vi "Navigation_Main_derping_stuff_up april 14.vi"() -> ()   [LabVIEW 2015]
uses:
  <vilib>/myRIO/Instrument Drivers/Onboard IO/PWM/typedefs/PWM Reference.ctl
  <vilib>/myRIO/Common/Instrument Driver Framework/Utilities/typedefs/myRIO Generic Hardware Reference.ctl
  <vilib>/myRIO/Common/Instrument Driver Framework/Utilities/typedefs/Hardware Version Enum.ctl
  <vilib>/myRIO/Common/Instrument Driver Framework/Utilities/typedefs/myRIO v1.0 Reference.ctl
  <vilib>/myRIO/Common/Instrument Driver Framework/Utilities/typedefs/Generic FPGA Reference.ctl
  <vilib>/myRIO/Common/Instrument Driver Framework/myRIO v1.0/PWM/typedefs/PWM Channels Enum.ctl
  <vilib>/myRIO/Instrument Drivers/Onboard IO/PWM/typedefs/PWM Configuration.ctl
  <vilib>/userdefined/High Color/nirio_resource_hc.ctl
  <vilib>/myRIO/Common/Instrument Driver Framework/myRIO v1.0/PWM/vis/myRIO v1.1 Open PWM.vi
  <vilib>/myRIO/Common/Instrument Driver Framework/Utilities/vis/Validate Channels.vi
  <vilib>/myRIO/Common/Instrument Driver Framework/myRIO v1.0/PWM/vis/myRIO v1.0 Reserve PWM.vi
  <vilib>/myRIO/Common/Instrument Driver Framework/myRIO v1.0/PWM/vis/myRIO v1.0 Build MUX Configuration PWM.vi
  <vilib>/myRIO/Common/Instrument Driver Framework/myRIO v1.0/Resource Manager/vis/myRIO v1.0 Reserve Channel List.vi
  <vilib>/myRIO/Common/Instrument Driver Framework/myRIO v1.0/Resource Manager/vis/myRIO v1.0 Create Configuration List.vi
  <vilib>/myRIO/Common/Instrument Driver Framework/myRIO v1.0/Resource Manager/vis/myRIO v1.0 Reserve Channel.vi
  <vilib>/myRIO/Common/Instrument Driver Framework/myRIO v1.0/Resource Manager/vis/myRIO v1.0 Unreserve Channel.vi
  <vilib>/myRIO/Common/Instrument Driver Framework/myRIO v1.0/Resource Manager/vis/myRIO v1.0 Build Mutex Name.vi
  <vilib>/FPGAPlugInAG/myRIO-1900/niLvFpga_Open_myRIO-1900.vi
  <vilib>/rvi/interface/common/dynamic/niFpgaDynamicAddResources.vi
  <vilib>/myRIO/Common/Instrument Driver Framework/Utilities/vis/FPGA Ref Manager.vi
  <vilib>/Utility/error.llb/Error Cluster From Error Code.vi
  <vilib>/myRIO/Common/Instrument Driver Framework/Utilities/vis/Ref Counter.vi
  <vilib>/rvi/errors/niLvFpgaAdjustHostInterfaceError.vi
  <vilib>/Utility/VariantDataType/GetNumericInfo.vi
  <vilib>/myRIO/Common/Instrument Driver Framework/myRIO v1.0/myRIO v1.1 Open.vi
  <vilib>/myRIO/Common/Instrument Driver Framework/Utilities/vis/IO Manager.vi
  <vilib>/myRIO/Common/Instrument Driver Framework/Utilities/vis/Configuration Manager.vi
  <vilib>/myRIO/Common/Instrument Driver Framework/myRIO v1.0/Resource Manager/vis/myRIO v1.0 Configure IO.vi
  <vilib>/myRIO/Common/Instrument Driver Framework/myRIO v1.0/myRIO v1.0 Close.vi
  <vilib>/myRIO/Common/Instrument Driver Framework/myRIO v1.0/PWM/vis/myRIO v1.0 Write PWM.vi
  <vilib>/addons/control/pid/pid.llb/PID (DBL).vi
  <vilib>/rvi/interface/nirviOpenFPGA/nirviOpenFPGA.xnode
  Navi/E/FPGA Bitfiles/NavigationProjec_FPGATarget2_FPGAMainNavigati_PWPHW8gwDxI.lvbitx
  <vilib>/rvi/interface/nirviReadWriteControl/nirviReadWriteControl.xnode
  <vilib>/myRIO/Instrument Drivers/Onboard IO/PWM/vis/myRIO PWM Open.xnode
  <vilib>/myRIO/Instrument Drivers/Onboard IO/PWM/PWM.lvlib
  <vilib>/myRIO/Instrument Drivers/Utilities/Utilities.lvlib
  NiFpgaLv.dll
  <vilib>/rvi/interface/Simulation/niFpgaSimulationCallBeginRW.vi
  <vilib>/addons/control/pid/NI_PID_pid.lvlib
panel:
  out "distance to goal":dbl
  out "loc_y":dbl
  out "loc_x":dbl
  out "loc_theta":dbl
  out "start y":dbl
  out "start angle":dbl=1.0
  out "start x":dbl=1.0
  in  "set start position":bool=TRUE
  out "goal reached":bool=TRUE
  out "x/y":dbl
  out "scale":dbl=1.0
  in  "x goal":dbl=10.0
  in  "L Desired Input Velocity (ft/s) 4":dbl(knob) scale=-4.0..4.0
  in  "R Min Linear Velocity (ft/s)  2":dbl=-2.0 format="%#_13g"
  in  "L Min Linear Velocity (ft/s) 9":dbl=-2.0 format="%#_13g"
  in  "R Max Linear Velocity (ft/s) 5":dbl=2.0 format="%#_13g"
  in  "L Max Linear Velocity (ft/s) 5":dbl=2.0 format="%#_13g"
  in  "R Desired Input Velocity (ft/s) 5":dbl(knob) scale=-4.0..4.0
  out "left":dbl
  out "right":dbl
  out "left wheels actual pwm":dbl
  in  "stop 3":bool
  out "left pwm":dbl(graph)
  out "dt out (s) 3":dbl format="%.3f"
  in  "output range 3":cluster{"output high":dbl, "output low":dbl}={"output high"=0.13333, "output low"=-0.13333} {"output low" format="%.6f"; "output high" format="%.5f"}
  in  "PID gains 3":T1={"proportional gain (Kc)"=0.002, "integral time (Ti, min)"=7e-07, "derivative time (Td, min)"=0.0} {"derivative time (Td, min)" format="%.8f"; "integral time (Ti, min)" format="%.8f"; "proportional gain (Kc)" format="%.8f"}
  out "desired pwm 2":dbl
  out "feedback 2":dbl
  out ".not. x? 3":bool
  out "Elapsed Time (s) 2":dbl caption="Elapsed Time (s)"
  out "x traveled 2":dbl
  out "y traveled 2":dbl
  out "avg 124":dbl
  out "avg 457":dbl
  out "psi dot 2":dbl
  out "distance traveled 2":dbl
  out "y dot 2":dbl
  out "x dot 2":dbl
  out "x position 2":dbl
  out "y position 2":dbl
  out "reset x y 2":dbl
  out "Tick Count(mSec) 2":u32 caption="Tick Count(mSec)"
  in  "start y 2":dbl=3.0
  in  "start x 2":dbl=1.0
  out "right wheels actual pwm":dbl
  in  "stop 2":bool
  out "right pwm":dbl(graph)
  out "dt out (s) 2":dbl format="%.3f"
  in  "output range 2":cluster{"output high":dbl, "output low":dbl}={"output high"=0.13333, "output low"=-0.13333} {"output low" format="%.6f"; "output high" format="%.5f"}
  in  "PID gains 2":T1={"proportional gain (Kc)"=0.002, "integral time (Ti, min)"=7e-07, "derivative time (Td, min)"=0.0} {"derivative time (Td, min)" format="%.8f"; "integral time (Ti, min)" format="%.8f"; "proportional gain (Kc)" format="%.8f"}
  out "desired pwm":dbl
  out "feedback":dbl
  out ".not. x? 2":bool
  out "Elapsed Time (s)":dbl
  out "LF Rot Velocity (rot/s)":dbl
  out "LM Rot Velocity (rot/s)":dbl
  out "LR Rot Velocity (rot/s)":dbl
  out "RR Rot Velocity (rot/s)":dbl
  out "RM Linear Velocity (rot/s)":dbl
  out "RF Linear Velocity (rot/s)":dbl
  in  "Encoder Reset":bool
  out "SYS.SELECTA":u8 format="%08b"
  out "ENC.B_c.CNTR":i32
  out "ENC.B_b.CNTR":i32
  out "ENC.B_a.CNTR":i32
  out "ENC.A_c.CNTR":i32
  out "ENC.A_b.CNTR":i32
  out "ENC.A_a.CNTR":i32
  in  "R Min Linear Velocity (ft/s)":dbl=-2.0 format="%#_13g"
  in  "R Max Linear Velocity (ft/s)":dbl=2.0 format="%#_13g"
  in  "L Min Linear Velocity (ft/s)":dbl=-2.0 format="%#_13g"
  in  "L Max Linear Velocity (ft/s)":dbl=2.0 format="%#_13g"
  out "Current Rot Velocity (rot/s)":T2(graph)
  # "Motor Control Parameters"
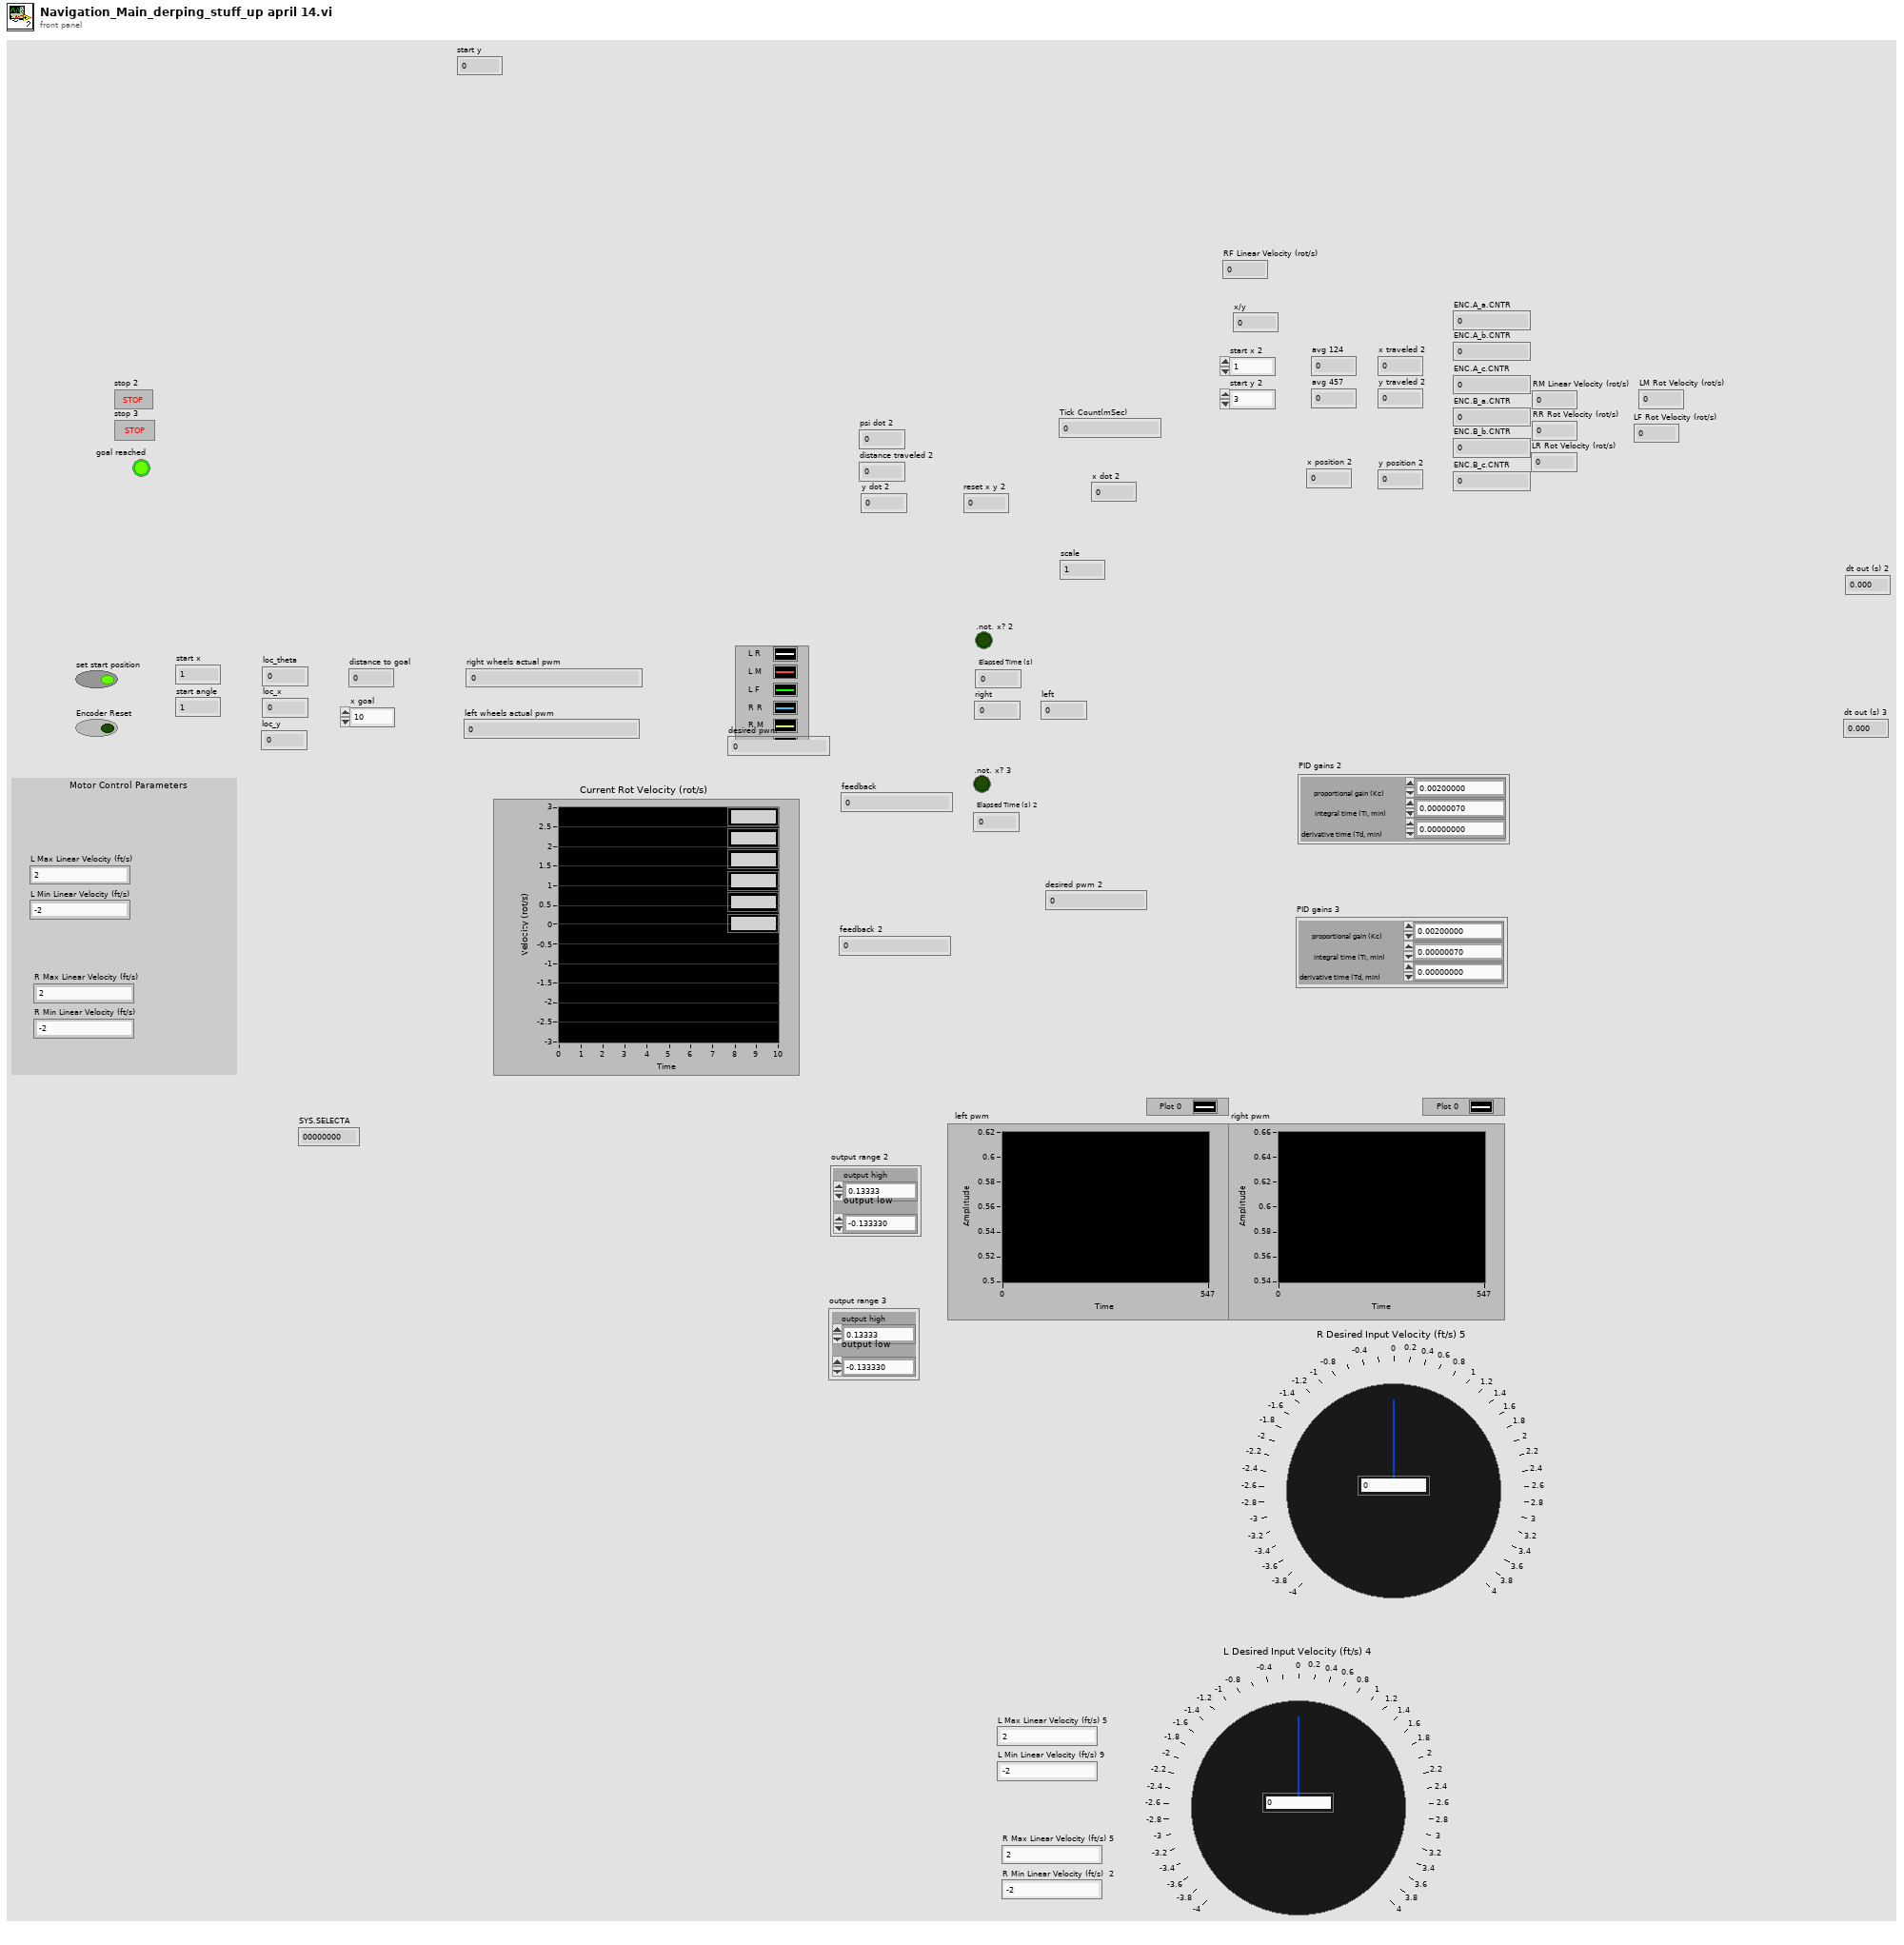
[diagram p1: front panel]
types:
  T1 = cluster{"proportional gain (Kc)":dbl, "integral time (Ti, min)":dbl, "derivative time (Td, min)":dbl}
  T2 = cluster{"Rotational Velocity (RPS)":dbl, "Rotational Velocity (RPS)":dbl, "Rotational Velocity (RPS)":dbl, "Rotational Velocity (RPS)":dbl, "Rotational Velocity (RPS)":dbl, "Rotational Velocity (RPS)":dbl}
  T3 = typedef "nirio_resource_hc.ctl" = tag
  T4 = typedef "Hardware Version Enum.ctl" = enum16{"Unknown", "myRIO-1900", "myRIO-1950", "roboRIO"}
  T5 = typedef "PWM.lvlib/PWM Reference.ctl" = cluster{"myRIO Reference":T6, "PWM Channels Enum":T9, "PWM Configuration":T10}
  T6 = typedef "myRIO Generic Hardware Reference.ctl" = cluster{"myRIO Model":T4, "myRIO Hardware Reference":T7}
  T7 = typedef "myRIO v1.0 Reference.ctl" = cluster{"Generic FPGA Reference":T8, "Allow multiple opens":bool}
  T8 = typedef "Generic FPGA Reference.ctl" = refnum<k20>
  T9 = typedef "PWM Channels Enum.ctl" = enum16{"Not Connected", "C/PWM0", "C/PWM1", "A/PWM0", "A/PWM1", "A/PWM2", "B/PWM0", "B/PWM1", "B/PWM2", "PWM/PWM0", "PWM/PWM1", "PWM/PWM2", "PWM/PWM3", "PWM/PWM4", "PWM/PWM5", "PWM/PWM6", "PWM/PWM7", "PWM/PWM8", "PWM/PWM9"}
  T10 = typedef "PWM.lvlib/PWM Configuration.ctl" = cluster{"Frequency":dbl, "Duty Cycle":dbl}
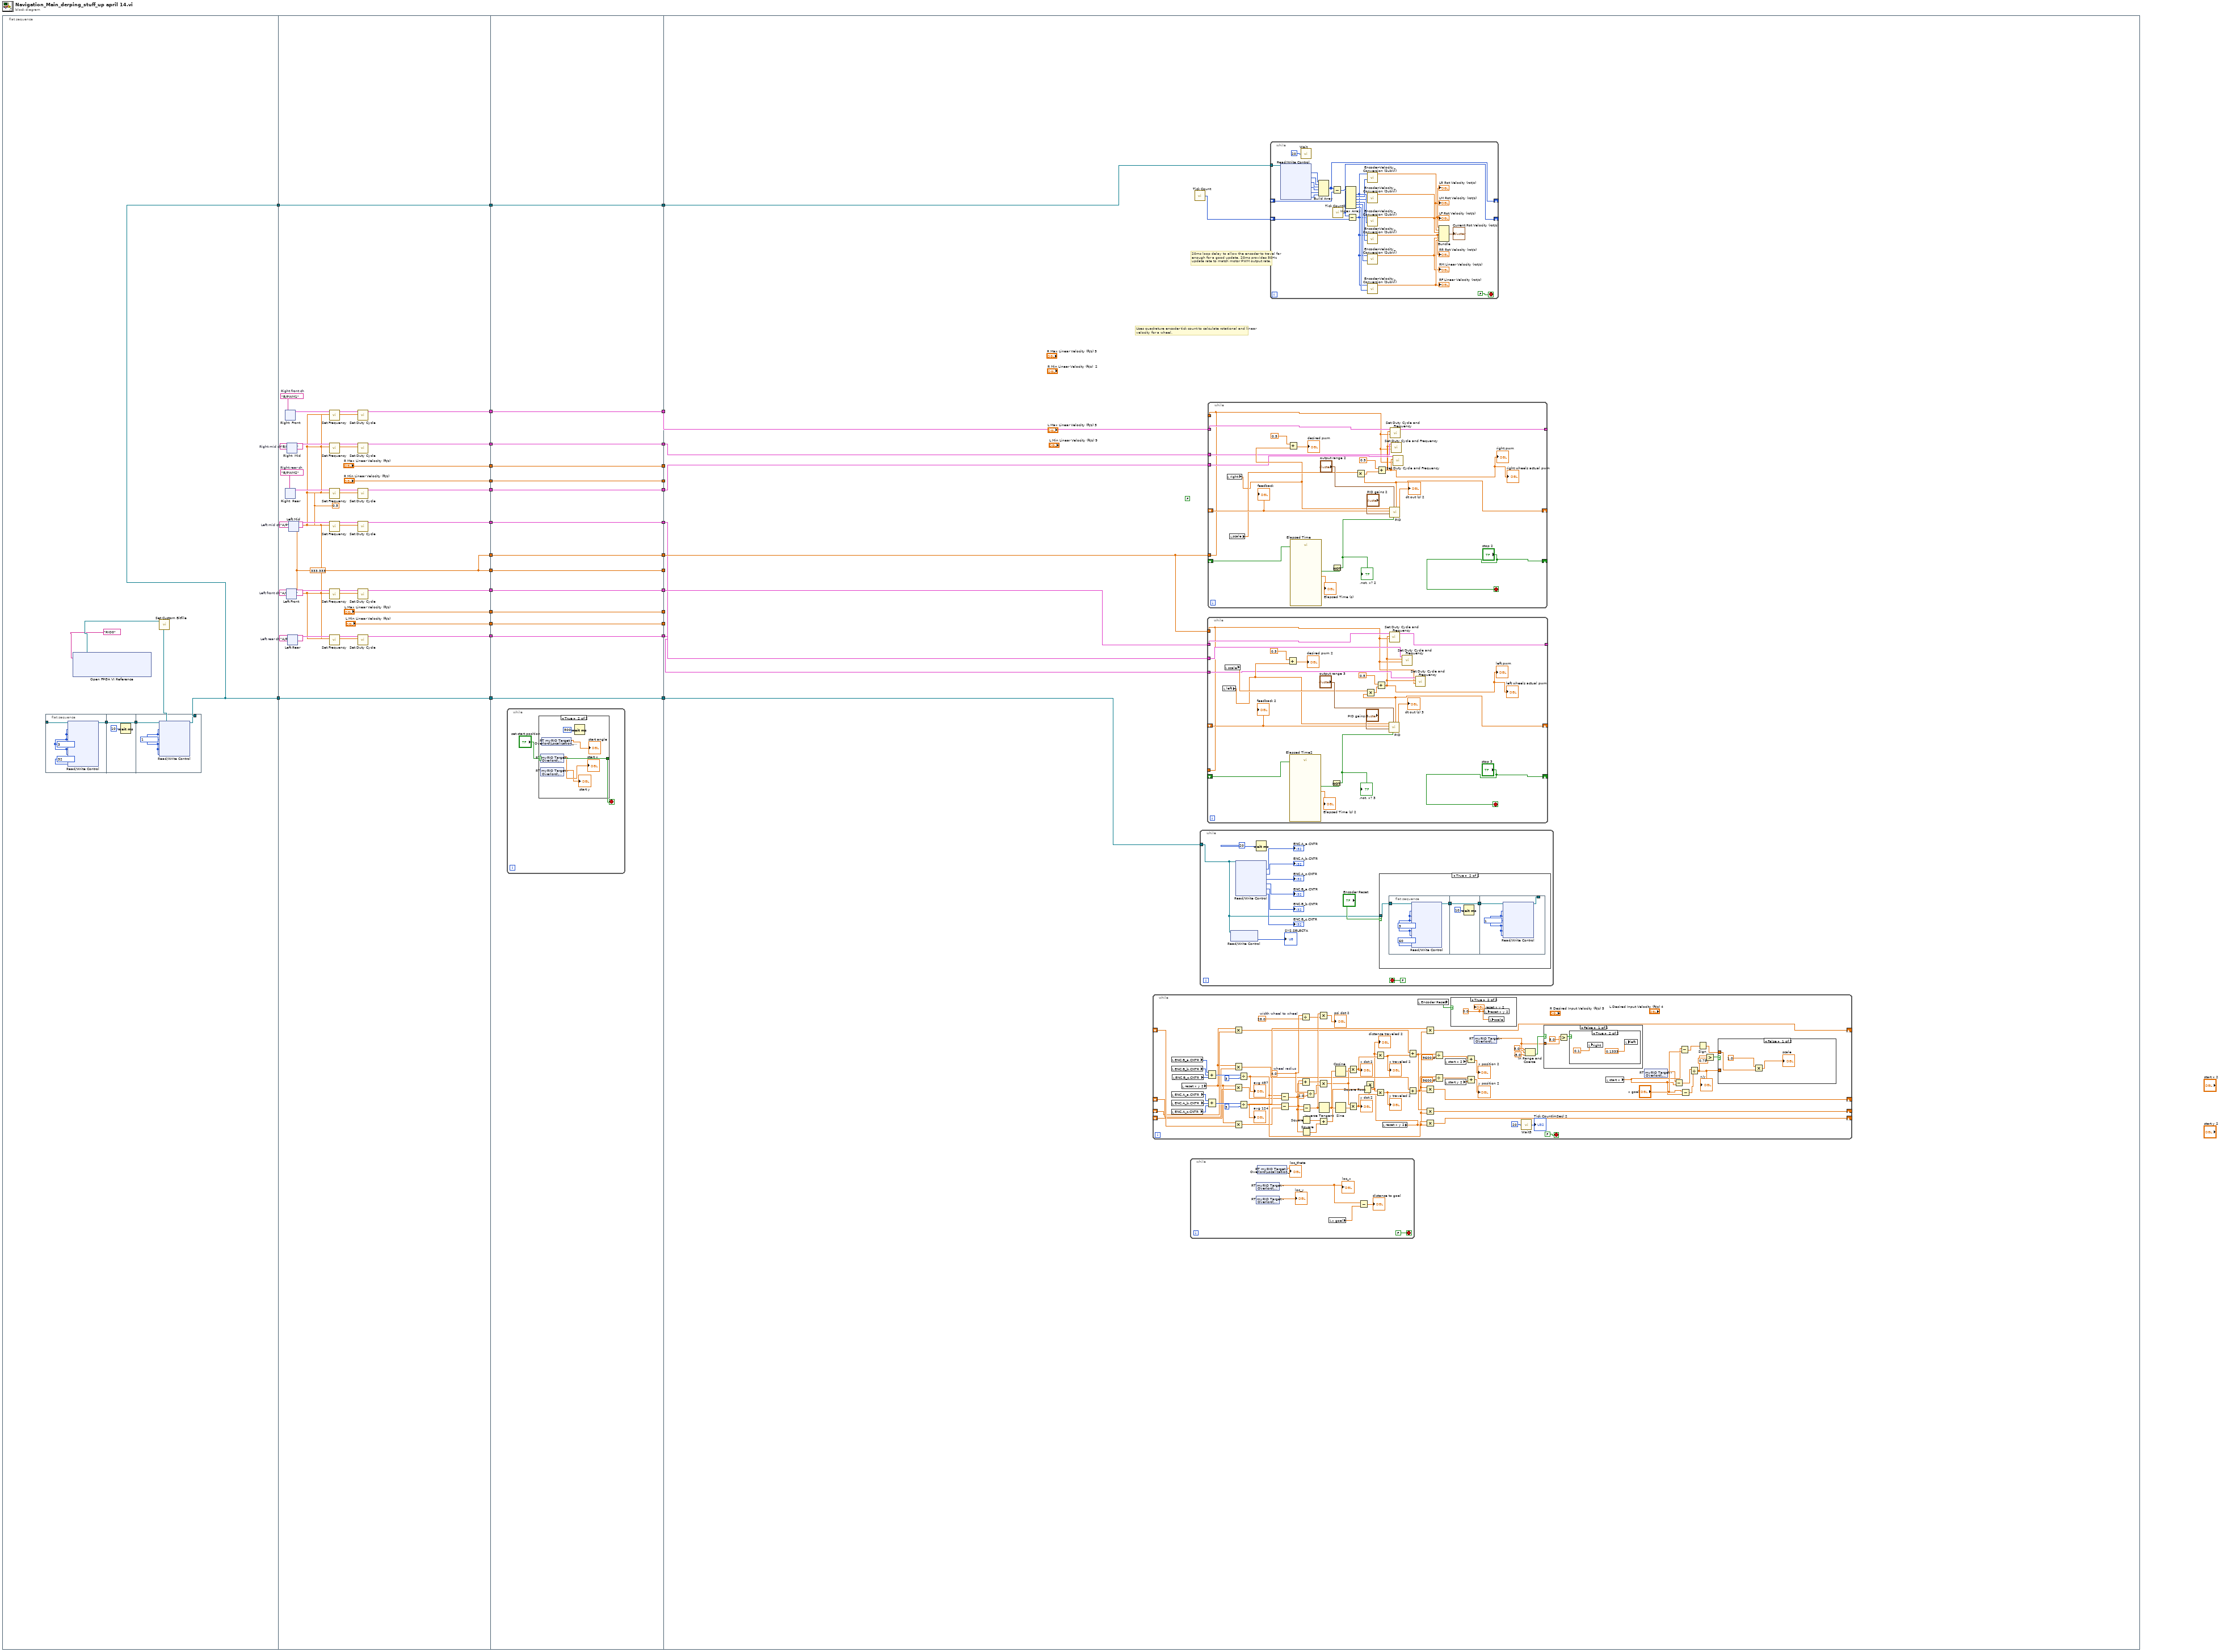
[diagram p0: block diagram]
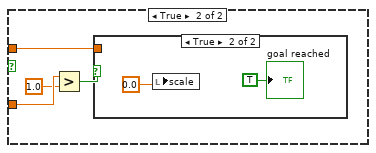
[diagram p3: hidden frame]
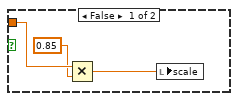
[diagram p4: hidden frame]
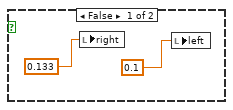
[diagram p5: hidden frame]
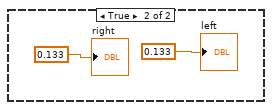
[diagram p6: hidden frame]
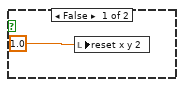
[diagram p7: hidden frame]
diagram:
  n1 = flat-sequence {
    tunnel: [w33] -> w30
    tunnel: [w33] -> w29
    tunnel: [w46] -> w28
    tunnel: [w61] -> w26
    tunnel: [w57] -> w24
    tunnel: [w56] -> w22
    tunnel: [w55] -> w20
    tunnel: [w54] -> w18
    tunnel: [w53] -> w16
    tunnel: ["L Max Linear Velocity (ft/s)"] -> w14
    tunnel: ["L Min Linear Velocity (ft/s)"] -> w12
    tunnel: ["R Max Linear Velocity (ft/s)"] -> w10
    tunnel: ["R Min Linear Velocity (ft/s)"] -> w8
    tunnel: [w48] -> w6
    tunnel: w30 -> [w47]
    tunnel: [w47] -> w4
    tunnel: w29 -> [w48]
    tunnel: [w46] -> w2
    tunnel: w28 -> [w187]
    tunnel: [w187] -> w27
    tunnel: w26 -> [w186]
    tunnel: [w186] -> w25
    tunnel: w24 -> [w185]
    tunnel: [w185] -> w23
    tunnel: w22 -> [w184]
    tunnel: [w184] -> w21
    tunnel: w20 -> [w183]
    tunnel: [w183] -> w19
    tunnel: w18 -> [w182]
    tunnel: [w182] -> w17
    tunnel: w16 -> [w181]
    tunnel: [w181] -> w15
    tunnel: w14 -> [w180]
    tunnel: [w180] -> w13
    tunnel: w12 -> [w179]
    tunnel: [w179] -> w11
    tunnel: w10 -> [w178]
    tunnel: [w178] -> w9
    tunnel: w8 -> [w177]
    tunnel: [w177] -> w7
    tunnel: w6 -> [w176]
    tunnel: [w176] -> w5
    tunnel: w4 -> [w175]
    tunnel: [w175] -> w3
    tunnel: w2 -> [w174]
    tunnel: [w174] -> w1
    tunnel: w27 -> [_]
    tunnel: w25 -> [w195]
    tunnel: w23 -> [w201]
    tunnel: w21 -> [w198]
    tunnel: w19 -> [w197]
    tunnel: w17 -> [w196]
    tunnel: w15 -> [w200]
    tunnel: w13 -> [_]
    tunnel: w11 -> [_]
    tunnel: w9 -> [_]
    tunnel: w7 -> [_]
    tunnel: w5 -> [w203]
    tunnel: w3 -> [w202]
    tunnel: w1 -> [w199]
    frame #0 {
      n2 = flat-sequence {
        tunnel: w34 -> [w39]
        tunnel: [w37] -> w36
        tunnel: w36 -> [w41]
        tunnel: [w41] -> w35
        tunnel: w35 -> [w44]
        tunnel: [w43] -> w33
        frame #0 {
          w38 = u8 32 ("SYS.SELECTA")
          w40 = u8 3 ("ENC.B_c.CNFG")
          n3 = xnode "Read/Write Control"("FPGA VI Reference In"=w39, "ENC.A_a.CNFG"=w40, "ENC.A_b.CNFG"=w40, "ENC.A_c.CNFG"=w40, "ENC.B_a.CNFG"=w40, "ENC.B_b.CNFG"=w40, "ENC.B_c.CNFG"=w40, "SYS.SELECTA"=w38, "SYS.SELECTB"=w38) -> ("FPGA VI Reference Out"=w37:refnum<k20>)  [unwired: 1 in, 1 out]
        }
        frame #1 {
          n4 = Wait (ms)(milliseconds to wait=u32 10) -> ()  [unwired: 1 out]
        }
        frame #2 {
          w45 = u8 1 ("ENC.B_c.CNFG")
          n5 = xnode "Read/Write Control"("FPGA VI Reference In"=w44, "ENC.A_a.CNFG"=w45, "ENC.A_b.CNFG"=w45, "ENC.A_c.CNFG"=w45, "ENC.B_a.CNFG"=w45, "ENC.B_b.CNFG"=w45, "ENC.B_c.CNFG"=w45) -> ("FPGA VI Reference Out"=w43:refnum<k20>)  [unwired: 1 in, 1 out]
        }
      }
      n6 = xnode "Open FPGA VI Reference"("resource name"=tag "RIO0") -> ("FPGA VI Reference Out"=w32:refnum<k20>)  [unwired: 1 in, 1 out]
      n7 = call <vilib>:"Set Custom Bitfile.vi"("Custom FPGA Reference In"=w32) -> ("Custom FPGA Reference Out"=w34:refnum<k20>)  [unwired: 9 in, 1 out]
    }
    frame #1 {
      w58 = 0.5 ("Duty Cycle")
      w46 = 333.333 ("Frequency [Hz]")
      w72 = tag "B/PWM2"  # Right rear ch
      w73 = tag "B/PWM0"  # Right mid ch
      w74 = tag "B/PWM1"  # Right front ch
      w75 = tag "A/PWM2"  # Left rear ch
      w76 = tag "A/PWM1"  # Left mid ch
      w77 = tag "A/PWM0"  # Left front ch
      n8 = xnode "Right  Front"("Channel Name"=w74) -> ("PWM Ref Out"=w68:T5)  [unwired: 2 in, 1 out]
      n9 = xnode "Right  Rear"("Channel Name"=w72) -> ("PWM Ref Out"=w66:T5)  [unwired: 2 in, 1 out]
      n10 = xnode "Left Front"("Channel Name"=w77) -> ("PWM Ref Out"=w71:T5)  [unwired: 2 in, 1 out]
      n11 = xnode "Right  Mid"("Channel Name"=w73) -> ("PWM Ref Out"=w67:T5)  [unwired: 2 in, 1 out]
      n12 = xnode "Left Rear"("Channel Name"=w75) -> ("PWM Ref Out"=w69:T5)  [unwired: 2 in, 1 out]
      n13 = xnode "Left Mid"("Channel Name"=w76) -> ("PWM Ref Out"=w70:T5)  [unwired: 2 in, 1 out]
      n14 = call <vilib>:"Set Frequency.vi"("Frequency [Hz]"=w46, "PWM Ref In"=w68) -> ("PWM Ref Out"=w62:T5)  [unwired: 7 in, 1 out]
      n15 = call <vilib>:"Set Frequency.vi"("Frequency [Hz]"=w46, "PWM Ref In"=w67) -> ("PWM Ref Out"=w63:T5)  [unwired: 7 in, 1 out]
      n16 = call <vilib>:"Set Frequency.vi"("Frequency [Hz]"=w46, "PWM Ref In"=w66) -> ("PWM Ref Out"=w64:T5)  [unwired: 7 in, 1 out]
      n17 = call <vilib>:"Set Frequency.vi"("Frequency [Hz]"=w46, "PWM Ref In"=w70) -> ("PWM Ref Out"=w59:T5)  [unwired: 7 in, 1 out]
      n18 = call <vilib>:"Set Frequency.vi"("Frequency [Hz]"=w46, "PWM Ref In"=w71) -> ("PWM Ref Out"=w65:T5)  [unwired: 7 in, 1 out]
      n19 = call <vilib>:"Set Frequency.vi"("Frequency [Hz]"=w46, "PWM Ref In"=w69) -> ("PWM Ref Out"=w60:T5)  [unwired: 7 in, 1 out]
      n20 = call <vilib>:"Set Duty Cycle.vi"("Duty Cycle"=w58, "PWM Ref In"=w62) -> ("PWM Ref Out"=w57:T5)  [unwired: 7 in, 1 out]
      n21 = call <vilib>:"Set Duty Cycle.vi"("Duty Cycle"=w58, "PWM Ref In"=w63) -> ("PWM Ref Out"=w56:T5)  [unwired: 7 in, 1 out]
      n22 = call <vilib>:"Set Duty Cycle.vi"("Duty Cycle"=w58, "PWM Ref In"=w64) -> ("PWM Ref Out"=w55:T5)  [unwired: 7 in, 1 out]
      n23 = call <vilib>:"Set Duty Cycle.vi"("Duty Cycle"=w58, "PWM Ref In"=w59) -> ("PWM Ref Out"=w54:T5)  [unwired: 7 in, 1 out]
      n24 = call <vilib>:"Set Duty Cycle.vi"("Duty Cycle"=w58, "PWM Ref In"=w65) -> ("PWM Ref Out"=w53:T5)  [unwired: 7 in, 1 out]
      n25 = call <vilib>:"Set Duty Cycle.vi"("Duty Cycle"=w58, "PWM Ref In"=w60) -> ("PWM Ref Out"=w61:T5)  [unwired: 7 in, 1 out]
    }
    frame #2 {
      n26 = while {
        stop <- w188 stop-if-true
        n27 = case shown="True" "set start position" {
          selector: "set start position" -> [_ w194]
          tunnel: [_ w194] -> w188
          frame False {
          }
          frame True {
            n28 = shared-variable "RT myRIO Target - Overlord\\Localization_Variables_r0.lvlib\\loc_x"() -> (→"start x":dbl)  [unwired: 1 in, 1 out]
            n29 = shared-variable "RT myRIO Target - Overlord\\Localization_Variables_r0.lvlib\\loc_y"() -> (→"start y":dbl)  [unwired: 1 in, 1 out]
            n30 = shared-variable "RT myRIO Target - Overlord\\Localization_Variables_r0.lvlib\\loc_theta"() -> (→"start angle":dbl)  [unwired: 1 in, 1 out]
            n31 = Wait (ms)(milliseconds to wait=u32 500) -> ()  [unwired: 1 out]
          }
        }
      }
    }
    frame #3 {
      (unwired) FALSE
      # "Uses quadrature encoder tick count to calculate rotational and linear velocity for a wheel."
      # "20ms loop delay to allow the encoder to travel far enough for a good update. 20ms provides 50Hz update rate to match motor PWM output rate."
      n32 = while {
        shift-right: [w258] -> _
        shift-left: _ -> [w296]
        shift-right: [w255] -> _
        shift-left: _ -> [w295]
        shift-right: [w257] -> _
        shift-left: _ -> [w270]
        shift-right: [w256] -> _
        shift-left: _ -> [w269]
        stop <- FALSE stop-if-true
        w291 = 28.0  # width wheel to wheel
        w292 = 4.0  # wheel radius
        n33 = local read "ENC.B_a.CNTR"() -> (w301:i32)
        n34 = local read "ENC.B_b.CNTR"() -> (w300:i32)
        n35 = local read "ENC.A_a.CNTR"() -> (w304:i32)
        n36 = local read "ENC.A_b.CNTR"() -> (w303:i32)
        n37 = local read "ENC.A_c.CNTR"() -> (w302:i32)
        n38 = local read "ENC.B_c.CNTR"() -> (w299:i32)
        n39 = local read "reset x y 2"() -> (w254:dbl)
        n40 = Compound Arithmetic op=ADD(w301, w300, w299) -> (w307:i32)
        n41 = Compound Arithmetic op=ADD(w304, w303, w302) -> (w308:i32)
        n42 = Multiply(x=w254, y=w269) -> (x*y=w260:dbl)
        n43 = Multiply(x=w254, y=w270) -> (x*y=w261:dbl)
        n44 = Multiply(x=w254, y=w295) -> (x*y=w259:dbl)
        n45 = Multiply(x=w254, y=w296) -> (x*y=w262:dbl)
        n46 = Divide(x=w307, y=3) -> (x/y=w294:dbl)
        "avg 457" <- w294
        n47 = Divide(x=w308, y=3) -> (x/y=w297:dbl)
        "avg 124" <- w297
        n48 = Subtract(x=w294, y=w259) -> (x-y=w284:dbl)
        n49 = Subtract(x=w297, y=w262) -> (x-y=w285:dbl)
        n50 = Divide(x=w292, y=w291) -> (x/y=w287:dbl)
        n51 = Add(x=w285, y=w284) -> (x+y=w289:dbl)
        n52 = Square(x=w285) -> (x^2=w282:dbl)
        n53 = Square(x=w284) -> (x^2=w283:dbl)
        n54 = Subtract(x=w285, y=w284) -> (x-y=w288:dbl)
        n55 = Divide(x=w292, y=2.0) -> (x/y=w290:dbl)
        n56 = Multiply(x=w288, y=w287) -> (x*y=→"psi dot 2":dbl)
        n57 = Multiply(x=w289, y=w290) -> (x*y=w278:dbl)
        n58 = Add(x=w282, y=w283) -> (x+y=w281:dbl)
        n59 = Inverse Tangent(1:w288) -> (0:w286:dbl)
        n60 = Cosine(x=w286) -> (cos(x)=w279:dbl)
        n61 = Sine(x=w286) -> (sin(x)=w280:dbl)
        n62 = Multiply(x=w278, y=w279) -> (x*y=w276:dbl)
        "x dot 2" <- w276
        n63 = Multiply(x=w278, y=w280) -> (x*y=w277:dbl)
        "y dot 2" <- w277
        n64 = Square Root(x=w281) -> (sqrt(x)=w275:dbl)
        n65 = local read "reset x y 2"() -> (w252:dbl)
        n66 = Multiply(x=w275, y=w252) -> (x*y=w253:dbl)
        "distance traveled 2" <- w253
        n67 = Multiply(x=w253, y=w276) -> (x*y=w274:dbl)
        "x traveled 2" <- w274
        n68 = Multiply(x=w253, y=w277) -> (x*y=w273:dbl)
        "y traveled 2" <- w273
        n69 = Add(x=w260, y=w274) -> (x+y=w272:dbl)
        n70 = Add(x=w261, y=w273) -> (x+y=w264:dbl)
        n71 = local read "Encoder Reset"() -> (w251:bool)
        n72 = Multiply(x=w297, y=w252) -> (x*y=w258:dbl)
        n73 = Multiply(x=w252, y=w264) -> (x*y=w257:dbl)
        n74 = Multiply(x=w272, y=w252) -> (x*y=w256:dbl)
        n75 = Multiply(x=w294, y=w252) -> (x*y=w255:dbl)
        n76 = Divide(x=w272, y=9600.0) -> (x/y=w267:dbl)
        n77 = Divide(x=w264, y=9600.0) -> (x/y=w268:dbl)
        n78 = local read "start x 2"() -> (w265:dbl)
        n79 = local read "start y 2"() -> (w266:dbl)
        n80 = case shown="True" w251 {
          frame False {
            n81 = local write "reset x y 2"(1.0) -> ()
          }
          frame True {
            w332 = 0.0
            n82 = local write "reset x y 2"(w332) -> ()
            n83 = local write "scale"(w332) -> ()
            "reset x y 2" <- w332
          }
        }
        n84 = Add(x=w267, y=w265) -> (x+y=→"x position 2":dbl)
        n85 = Add(x=w268, y=w266) -> (x+y=→"y position 2":dbl)
        n86 = shared-variable "RT myRIO Target - Overlord\\Localization_Variables_r0.lvlib\\loc_x"() -> (w234:dbl)  [unwired: 1 in, 1 out]
        n87 = call "Wait3"("Count(mSec)"=u32 20) -> ("Tick Count(mSec)"=→"Tick Count(mSec) 2":u32)
        n88 = In Range and Coerce(upper limit=5.0, x=w234, lower limit=-5.0) -> (In Range?=w245:bool)  [unwired: 1 out]
        n89 = case shown="False" w245 {
          tunnel: w234 -> [w324 _]
          frame False {
            n90 = Greater?(x=w324, y=5.0) -> (0:w322:bool)
            n91 = case shown="True" w322 {
              frame False {
                n92 = local write "right"(0.133) -> ()
                n93 = local write "left"(0.1) -> ()
              }
              frame True {
                n94 = local write "right"(0.1) -> ()
                n95 = local write "left"(0.1333) -> ()
              }
            }
          }
          frame True {
            "right" <- 0.133
            "left" <- 0.133
          }
        }
        n96 = local read "start x"() -> (w236:dbl)
        n97 = shared-variable "RT myRIO Target - Overlord\\Localization_Variables_r0.lvlib\\loc_x"() -> (w233:dbl)  [unwired: 1 in, 1 out]
        n98 = Subtract(x=w233, y=w236) -> (x-y=w241:dbl)
        n99 = Subtract(x=w236, y="x goal") -> (x-y=w238:dbl)
        n100 = Subtract(x="x goal", y=w236) -> (x-y=w240:dbl)
        n101 = Divide(x=w241, y=w240) -> (x/y=w242:dbl)
        "x/y" <- w242
        n102 = Sign(1:w238) -> (0:w237:dbl)
        n103 = Greater?(x=w242, y=0.75) -> (0:w243:bool)
        n104 = case shown="False" w243 {
          tunnel: w242 -> [_ w316]
          tunnel: w237 -> [w311 w313]
          frame False {
            n105 = Multiply(x=1.0, y=w311) -> (x*y=→"scale":dbl)
          }
          frame True {
            n106 = Greater?(x=w316, y=1.0) -> (0:w314:bool)
            n107 = case shown="True" w314 {
              tunnel: w313 -> [w319 _]
              frame False {
                n108 = Multiply(x=w319, y=0.85) -> (x*y=w317:dbl)
                n109 = local write "scale"(w317) -> ()
              }
              frame True {
                n110 = local write "scale"(0.0) -> ()
                "goal reached" <- TRUE
              }
            }
          }
        }
      }
      n111 = while {
        stop <- FALSE stop-if-true
        n112 = shared-variable "RT myRIO Target - Overlord\\Localization_Variables_r0.lvlib\\loc_x"() -> (w208:dbl)  [unwired: 1 in, 1 out]
        "loc_x" <- w208
        n113 = shared-variable "RT myRIO Target - Overlord\\Localization_Variables_r0.lvlib\\loc_y"() -> (→"loc_y":dbl)  [unwired: 1 in, 1 out]
        n114 = shared-variable "RT myRIO Target - Overlord\\Localization_Variables_r0.lvlib\\loc_theta"() -> (→"loc_theta":dbl)  [unwired: 1 in, 1 out]
        n115 = local read "x goal"() -> (w207:dbl)
        n116 = Subtract(x=w208, y=w207) -> (x-y=→"distance to goal":dbl)
      }
      n117 = call "Tick Count"() -> ("Tick Count(uSec)"=w204:u32)
      n118 = while {
        tunnel: w203 -> [w355]
        stop <- FALSE stop-if-true
        n119 = xnode "Read/Write Control"("FPGA VI Reference In"=w355) -> ("SYS.SELECTA"=→"SYS.SELECTA":u8)  [unwired: 1 in, 2 out]
        n120 = xnode "Read/Write Control"("FPGA VI Reference In"=w355) -> ("ENC.A_a.CNTR"=→"ENC.A_a.CNTR":u32, "ENC.A_b.CNTR"=→"ENC.A_b.CNTR":u32, "ENC.A_c.CNTR"=→"ENC.A_c.CNTR":u32, "ENC.B_a.CNTR"=→"ENC.B_a.CNTR":u32, "ENC.B_b.CNTR"=→"ENC.B_b.CNTR":u32, "ENC.B_c.CNTR"=→"ENC.B_c.CNTR":u32)  [unwired: 1 in, 2 out]
        n121 = Wait (ms)(milliseconds to wait=u32 20) -> ()  [unwired: 1 out]
        n122 = case shown="True" "Encoder Reset" {
          tunnel: w355 -> [_ w366]
          frame False {
          }
          frame True {
            n123 = flat-sequence {
              tunnel: w366 -> [w371]
              tunnel: [w369] -> w368
              tunnel: w368 -> [w373]
              tunnel: [w373] -> w367
              tunnel: w367 -> [w376]
              tunnel: [w375] -> _
              frame #0 {
                w370 = u8 60 ("SYS.SELECTA")
                w372 = u8 3 ("ENC.B_c.CNFG")
                n124 = xnode "Read/Write Control"("FPGA VI Reference In"=w371, "ENC.A_a.CNFG"=w372, "ENC.A_b.CNFG"=w372, "ENC.A_c.CNFG"=w372, "ENC.B_a.CNFG"=w372, "ENC.B_b.CNFG"=w372, "ENC.B_c.CNFG"=w372, "SYS.SELECTA"=w370, "SYS.SELECTB"=w370) -> ("FPGA VI Reference Out"=w369:refnum<k20>)  [unwired: 1 in, 1 out]
              }
              frame #1 {
                n125 = Wait (ms)(milliseconds to wait=u32 10) -> ()  [unwired: 1 out]
              }
              frame #2 {
                w377 = u8 1 ("ENC.B_c.CNFG")
                n126 = xnode "Read/Write Control"("FPGA VI Reference In"=w376, "ENC.A_a.CNFG"=w377, "ENC.A_b.CNFG"=w377, "ENC.A_c.CNFG"=w377, "ENC.B_a.CNFG"=w377, "ENC.B_b.CNFG"=w377, "ENC.B_c.CNFG"=w377) -> ("FPGA VI Reference Out"=w375:refnum<k20>)  [unwired: 1 in, 1 out]
              }
            }
          }
        }
      }
      n127 = while {
        tunnel: w200 -> [w231]
        tunnel: [w232] -> _
        tunnel: w199 -> [w211]
        shift-right: [w217] -> _
        shift-left: _ -> [w227]
        shift-right: ["stop 3"] -> _
        shift-left: _ -> [w222]
        tunnel: [w211] -> _
        tunnel: w196 -> [w214]
        tunnel: w195 -> [w213]
        stop <- "stop 3" stop-if-true
        n128 = local read "left"() -> (w215:dbl)
        n129 = local read "scale"() -> (w218:dbl)
        n130 = Add(x=0.5, y=w215) -> (x+y=→"desired pwm 2":dbl)
        n131 = call "Elapsed Time2"("Reset"=w222) -> ("Elapsed Time (s)"=→"Elapsed Time (s) 2":dbl, "Time has Elapsed"=w225:bool)  [unwired: 11 in, 6 out]
        n132 = Not(x=w225) -> (.not. x?=w224:bool)
        ".not. x? 3" <- w224
        n133 = call-poly <vilib>:"PID.vi"("reinitialize? (F)"=w224, "output range"="output range 3", "PID gains"="PID gains 3", "process variable"=w227, "setpoint"=w215) -> ("dt out (s)"=→"dt out (s) 3":dbl, "output"=w217:dbl)  [unwired: 5 in]
        n134 = Multiply(x=w218, y=w217) -> (x*y=w216:dbl)
        n135 = Add(x=0.5, y=w216) -> (x+y=w212:dbl)
        "left wheels actual pwm" <- w212
        "left pwm" <- w212
        n136 = call <vilib>:"Set Duty Cycle and Frequency.vi"("Frequency [Hz]"=w211, "Duty Cycle"=w212, "PWM Ref In"=w231) -> ("PWM Ref Out"=w232:T5)  [unwired: 6 in, 1 out]
        n137 = call <vilib>:"Set Duty Cycle and Frequency.vi"("Frequency [Hz]"=w211, "Duty Cycle"=w212, "PWM Ref In"=w214) -> ()  [unwired: 6 in, 2 out]
        n138 = call <vilib>:"Set Duty Cycle and Frequency.vi"("Frequency [Hz]"=w211, "Duty Cycle"=w212, "PWM Ref In"=w213) -> ()  [unwired: 6 in, 2 out]
        "feedback 2" <- w227
      }
      n139 = while {
        tunnel: w201 -> [w353]
        tunnel: [w354] -> _
        tunnel: [w333] -> _
        shift-right: [w339] -> _
        shift-left: _ -> [w349]
        shift-right: ["stop 2"] -> _
        shift-left: _ -> [w344]
        tunnel: w199 -> [w333]
        tunnel: w198 -> [w336]
        tunnel: w197 -> [w335]
        stop <- "stop 2" stop-if-true
        n140 = local read "right"() -> (w337:dbl)
        n141 = local read "scale"() -> (w340:dbl)
        n142 = Add(x=0.5, y=w337) -> (x+y=→"desired pwm":dbl)
        n143 = call "Elapsed Time"("Reset"=w344) -> ("Elapsed Time (s)"=→"Elapsed Time (s)":dbl, "Time has Elapsed"=w347:bool)  [unwired: 11 in, 6 out]
        n144 = Not(x=w347) -> (.not. x?=w346:bool)
        ".not. x? 2" <- w346
        n145 = call-poly <vilib>:"PID.vi"("reinitialize? (F)"=w346, "output range"="output range 2", "PID gains"="PID gains 2", "process variable"=w349, "setpoint"=w337) -> ("dt out (s)"=→"dt out (s) 2":dbl, "output"=w339:dbl)  [unwired: 5 in]
        n146 = Multiply(x=w340, y=w339) -> (x*y=w338:dbl)
        n147 = Add(x=0.5, y=w338) -> (x+y=w334:dbl)
        "right wheels actual pwm" <- w334
        "right pwm" <- w334
        n148 = call <vilib>:"Set Duty Cycle and Frequency.vi"("Frequency [Hz]"=w333, "Duty Cycle"=w334, "PWM Ref In"=w353) -> ("PWM Ref Out"=w354:T5)  [unwired: 6 in, 1 out]
        n149 = call <vilib>:"Set Duty Cycle and Frequency.vi"("Frequency [Hz]"=w333, "Duty Cycle"=w334, "PWM Ref In"=w336) -> ()  [unwired: 6 in, 2 out]
        n150 = call <vilib>:"Set Duty Cycle and Frequency.vi"("Frequency [Hz]"=w333, "Duty Cycle"=w334, "PWM Ref In"=w335) -> ()  [unwired: 6 in, 2 out]
        "feedback" <- w349
      }
      n151 = while {
        shift-right: [w396] -> _
        shift-left: _ -> [w395]
        shift-right: [w393] -> _
        shift-left: w204 -> [w392]
        tunnel: w202 -> [w403]
        stop <- FALSE stop-if-true
        n152 = xnode "Read/Write Control"("FPGA VI Reference In"=w403) -> ("ENC.A_a.CNTR"=w402:u32, "ENC.A_b.CNTR"=w401:u32, "ENC.A_c.CNTR"=w400:u32, "ENC.B_a.CNTR"=w399:u32, "ENC.B_b.CNTR"=w398:u32, "ENC.B_c.CNTR"=w397:u32)  [unwired: 1 in, 2 out]
        n153 = call "Wait"("Count(mSec)"=u32 20) -> ()  [unwired: 1 out]
        n154 = Build Array(w402, w401, w400, w399, w398, w397) -> (w396:u32[])
        n155 = Subtract(x=w396, y=w395) -> (x-y=w394:u32[])
        n156 = call "Tick Count2"() -> ("Tick Count(uSec)"=w393:u32)
        n157 = Index Array(array=w394) -> (element #1=w391:u32, element #2=w390:u32, element #3=w389:u32, element #4=w388:u32, element #5=w387:u32, element #6=w386:u32)  [unwired: 6 in]
        n158 = Subtract(x=w393, y=w392) -> (x-y=w385:u32)
        n159 = call "Encoder-Velocity_Conversion (SubVI).vi"("delta  Encoder Count"=w390, "dt (uSec)"=w385) -> ("Rotational Velocity (RPS)"=w380:dbl)  [unwired: 7 in, 2 out]
        "LM Rot Velocity (rot/s)" <- w380
        n160 = call "Encoder-Velocity_Conversion (SubVI).vi"("delta  Encoder Count"=w389, "dt (uSec)"=w385) -> ("Rotational Velocity (RPS)"=w379:dbl)  [unwired: 7 in, 2 out]
        "LF Rot Velocity (rot/s)" <- w379
        n161 = call "Encoder-Velocity_Conversion (SubVI).vi"("delta  Encoder Count"=w391, "dt (uSec)"=w385) -> ("Rotational Velocity (RPS)"=w381:dbl)  [unwired: 7 in, 2 out]
        "LR Rot Velocity (rot/s)" <- w381
        n162 = call "Encoder-Velocity_Conversion (SubVI).vi"("delta  Encoder Count"=w388, "dt (uSec)"=w385) -> ("Rotational Velocity (RPS)"=w378:dbl)  [unwired: 7 in, 2 out]
        "RR Rot Velocity (rot/s)" <- w378
        n163 = call "Encoder-Velocity_Conversion (SubVI).vi"("delta  Encoder Count"=w387, "dt (uSec)"=w385) -> ("Rotational Velocity (RPS)"=w382:dbl)  [unwired: 7 in, 2 out]
        "RM Linear Velocity (rot/s)" <- w382
        n164 = call "Encoder-Velocity_Conversion (SubVI).vi"("delta  Encoder Count"=w386, "dt (uSec)"=w385) -> ("Rotational Velocity (RPS)"=w383:dbl)  [unwired: 7 in, 2 out]
        "RF Linear Velocity (rot/s)" <- w383
        n165 = Bundle("Rotational Velocity (RPS)"=w381, "Rotational Velocity (RPS)"=w380, "Rotational Velocity (RPS)"=w379, "Rotational Velocity (RPS)"=w378, "Rotational Velocity (RPS)"=w382, "Rotational Velocity (RPS)"=w383) -> (→"Current Rot Velocity (rot/s)":T2)  [unwired: 1 in]
      }
    }
  }
